vi "RPMToRawUnits-2048-CPR.vi"(2 "Gear Ratio":dbl=1.0, 3 "RPM":dbl) -> (0 "Raw Units":i32)   [LabVIEW 2020, in "TitanLib.lvlib"]
uses:
  TitanLib.lvlib
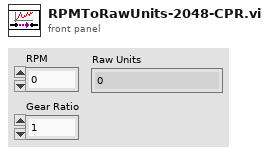
[diagram p1: front panel]
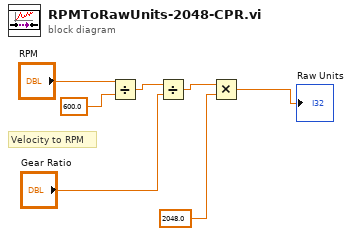
[diagram p0: block diagram]
diagram:
  # "Velocity to RPM"
  n1 = Divide(x="RPM", y=600.0) -> (x/y=w5:dbl)
  n2 = Divide(x=w5, y="Gear Ratio") -> (x/y=w3:dbl)
  n3 = Multiply(x=w3, y=2048.0) -> (x*y=→"Raw Units":dbl)
